vi "ukol1.vi"() -> ()   [LabVIEW 2023]
uses:
  <vilib>/Analysis/2dsp.llb/Real FFT.vi
  <vilib>/Analysis/NI_AALPro.lvlib
  <vilib>/measure/NI_MABase.lvlib
panel:
  out "XY Graph":cluster{dbl[], dbl[]}(graph)
  out "frekvence":dbl
  in  "Cluster 2":T1={"frequency"=10.0, "amplitude"=1.0, "phase"=0.0} {"phase" format="%.2p"; "amplitude" format="%0.2p"; "frequency" format="%0.2p"}
  in  "stop":bool
  out "Waveform Graph":waveform(dbl)(graph)
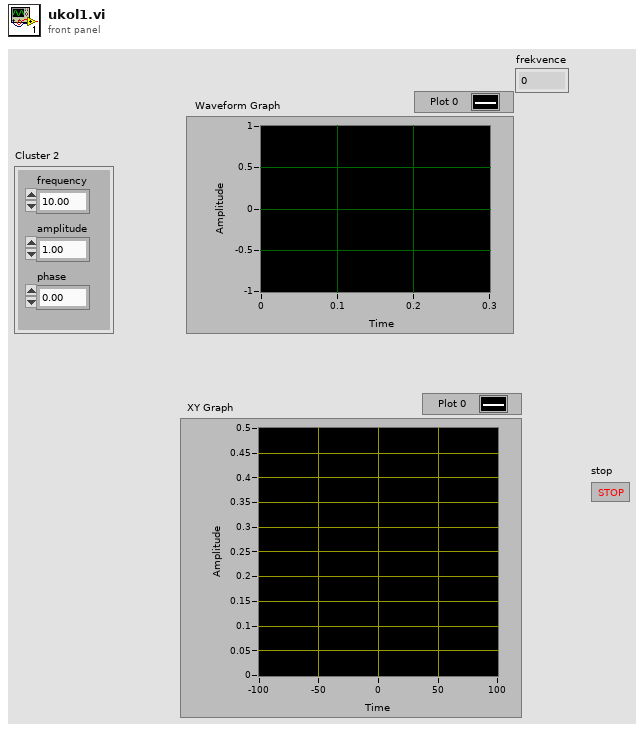
[diagram p1: front panel]
types:
  T1 = cluster{"frequency":dbl, "amplitude":dbl, "phase":dbl}
  T2 = cluster{"frequency":dbl, "amplitude":dbl, "phase":dbl}[]
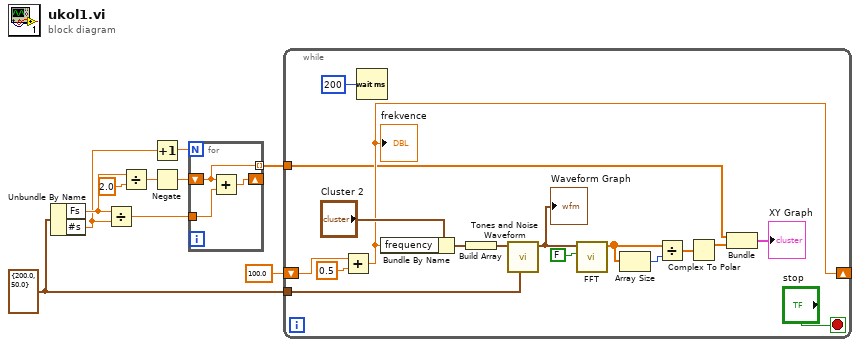
[diagram p0: block diagram]
diagram:
  w8 = cluster{"Fs":dbl, "#s":dbl} {"Fs"=200.0, "#s"=50.0} ("sampling info")
  n1 = Unbundle By Name(w8) -> ("Fs"=w5:dbl, "#s"=w3:dbl)
  n2 = Divide(x=w5, y=w3) -> (x/y=w4:dbl)
  n3 = Divide(x=w5, y=2.0) -> (x/y=w9:dbl)
  n4 = Increment(x=w3) -> (x+1=w2:dbl)
  n5 = Negate(x=w9) -> (-x=w7:dbl)
  n6 = for {
    N: w2 -> [_]
    shift-right: [w12] -> _
    shift-left: w7 -> [w11]
    tunnel: w4 -> [w13]
    tunnel: [w11] -> w1 mode=indexing
    n7 = Add(x=w11, y=w13) -> (x+y=w12:dbl)
  }
  n8 = while {
    shift-right: [w18] -> _
    shift-left: 100.0 -> [w29]
    tunnel: w8 -> [w17]
    tunnel: w1 -> [w14]
    stop <- "stop" stop-if-true
    n9 = Add(x=w29, y=0.5) -> (x+y=w18:dbl)
    "frekvence" <- w18
    n10 = Wait (ms)(milliseconds to wait=u32 200) -> ()  [unwired: 1 out]
    n11 = Bundle By Name(cluster="Cluster 2", "frequency"=w18) -> (w21:T1)
    n12 = Build Array(w21) -> (w20:T2)
    n13 = call <vilib>:"Tones and Noise Waveform.vi"("sampling info"=w17, "tones"=w20) -> ("signal out"=w22:waveform(dbl))  [unwired: 8 in, 1 out]
    "Waveform Graph" <- w22
    n14 = call-poly <vilib>:"FFT.vi"("shift?"=FALSE, "X"=w22) -> ("FFT {X}"=w25:cdb[])  [unwired: 8 in, 1 out]
    n15 = Array Size(array=w25) -> (size(s)=w24:i32)
    n16 = Divide(x=w25, y=w24) -> (x/y=w23:cdb[])
    n17 = Complex To Polar(r * e^(i*theta)=w23) -> (r=w15:dbl[])  [unwired: 1 out]
    n18 = Bundle(w14, w15) -> (→"XY Graph":cluster{dbl[], dbl[]})  [unwired: 1 in]
  }
